vi "EX 3.vi"() -> ()   [LabVIEW 2018]
panel:
  out "Led":bool
  out "Nom":string
  out "Prénom":string
  in  "Nom brut":string
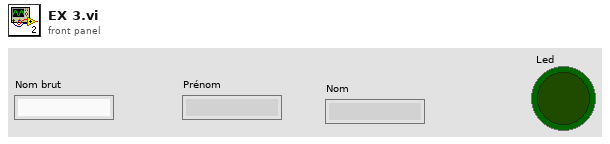
[diagram p1: front panel]
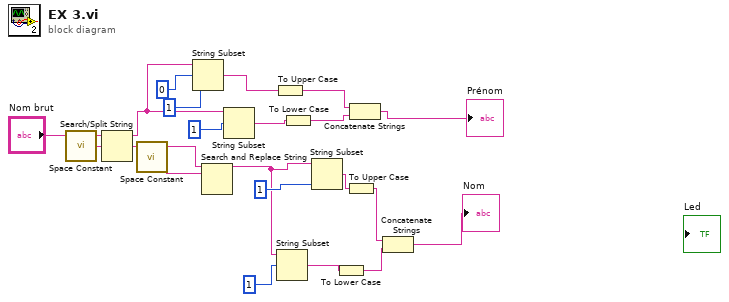
[diagram p0: block diagram]
diagram:
  n1 = call <vilib>:"Space Constant.vi"() -> ("String"=w20:string)
  n2 = Search/Split String(string="Nom brut", search string/char (-)=w20) -> (substring before match=w14:string, match + rest of string=w18:string)  [unwired: 1 in, 1 out]
  n3 = call <vilib>:"Space Constant.vi"() -> ("String"=w19:string)
  n4 = String Subset(string=w14, offset (0)=0, length (rest)=1) -> (substring=w15:string)
  n5 = Search and Replace String(input string=w18, search string=w19) -> (result string=w9:string)  [unwired: 6 in, 3 out]
  n6 = String Subset(string=w14, offset (0)=1) -> (substring=w4:string)  [unwired: 1 in]
  n7 = To Upper Case(1:w15) -> (0:w12:string)
  n8 = String Subset(string=w9, offset (0)=1) -> (substring=w2:string)  [unwired: 1 in]
  n9 = To Lower Case(string=w4) -> (all lower case string=w3:string)
  n10 = String Subset(string=w9, length (rest)=1) -> (substring=w10:string)  [unwired: 1 in]
  n11 = To Lower Case(string=w2) -> (all lower case string=w1:string)
  n12 = To Upper Case(1:w10) -> (0:w7:string)
  n13 = Concatenate Strings(w12, w3) -> (→"Prénom":string)
  n14 = Concatenate Strings(w7, w1) -> (→"Nom":string)
